vi "Present Data.vi"(8 "error in (no error)":errorcluster, 11 "List Seen Processes View Model In":refnum<class "List Box View Model.lvclass">) -> (0 "error out":errorcluster, 2 "Message List":string[](array[string]), 3 "List Seen Processes View Model Out":refnum<class "List Box View Model.lvclass">)   [LabVIEW 2020, in "List Box View Model.lvclass"]
uses:
  List Box View Model.lvclass
  List Box View Model.lvclass/List Box View Model.ctl
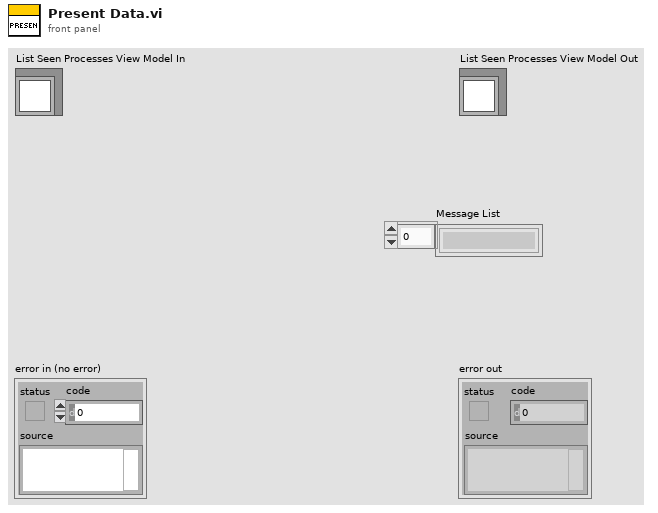
[diagram p1: front panel]
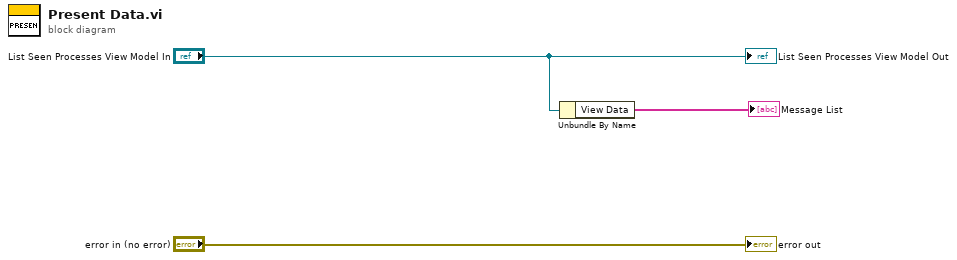
[diagram p0: block diagram]
diagram:
  n1 = Unbundle By Name("List Seen Processes View Model In") -> ("View Data"=→"Message List":string[])
  "error out" <- "error in (no error)"
  "List Seen Processes View Model Out" <- "List Seen Processes View Model In"
